vi "WAPIAerCheckInitz.vi"(3 "board":i16, 9 "error in (no error)":errorcluster) -> (0 "result":bool, 6 "error out":errorcluster)   [LabVIEW 2009]
uses:
  win50032.dll
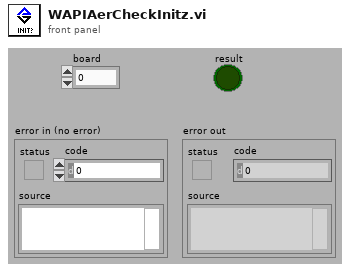
[diagram p1: front panel]
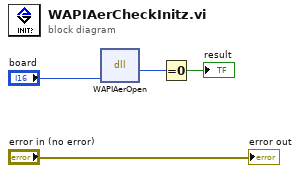
[diagram p0: block diagram]
diagram:
  n1 = dll-call lib="Win50032.dll" fn="WAPIAerOpen" label="WAPIAerCheckInitz"("board"="board") -> ("return type"=w2:u32)  [unwired: 4 in, 2 out]
  n2 = Equal To 0?(x=w2) -> (x = 0?=→"result":bool)
  "error out" <- "error in (no error)"
